vi "Latch Data.vi"(8 "error in (no error)":errorcluster, 10 "Time Stamp":timestamp=timestamp(3631881134.247515 s since 1904-01-01), 11 "dt":dbl=2000.0) -> (0 "error out":errorcluster, 3 "Waveform Array":waveform(dbl)[](array[waveform])=[{"t0"=timestamp(3631881134.247515 s since 1904-01-01), "dt"=2000.0, "Y"=[0.0], "attributes"=variant("NI_ChannelName"=variant(string "Pump 1 Flow"))}])   [LabVIEW 2018, in "CSV Log.lvlib"]
uses:
  CSV Log.lvlib
  <vilib>/ptbypt/NI_PtbyPt.lvlib
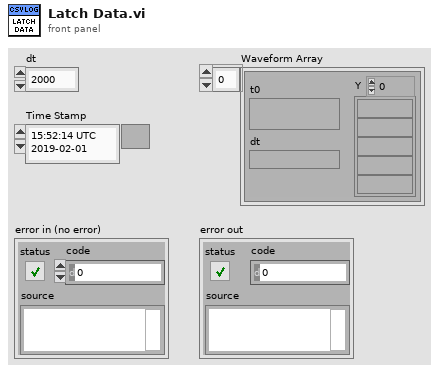
[diagram p1: front panel]
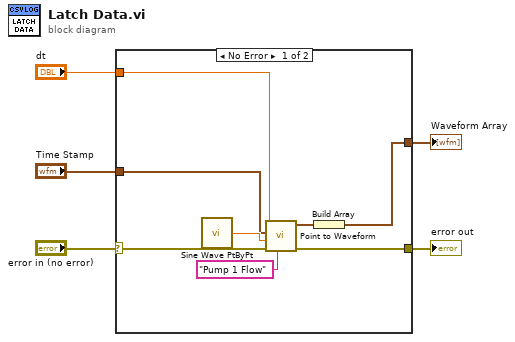
[diagram p0: block diagram]
diagram:
  n1 = case shown="No Error" "error in (no error)" {
    selector: "error in (no error)" -> [w6 w14]
    tunnel: [w13 _] -> w5
    tunnel: [w11 w14] -> w4
    tunnel: "dt" -> [w8 _]
    tunnel: "Time Stamp" -> [w7 _]
    frame No Error {
      n2 = call <vilib>:"Sine Wave PtByPt.vi"() -> ("sine wave"=w9:dbl)  [unwired: 4 in]
      n3 = call "Point to Waveform.vi"("Channel name"="Pump 1 Flow", "error in (no error)"=w6, "data"=w9, "Time Stamp"=w7, "dt"=w8) -> ("error out"=w11:errorcluster, "Waveform"=w12:waveform(dbl))  [unwired: 5 in]
      n4 = Build Array(w12) -> (w13:waveform(dbl)[])
    }
    frame Error {
    }
  }
  "Waveform Array" <- w5
  "error out" <- w4
